vi "Edit Documentation of Properties.vi"   [LabVIEW 2015]
uses:
  Project Manipulation Scripts/Project Manipulation Scripts.lvlib
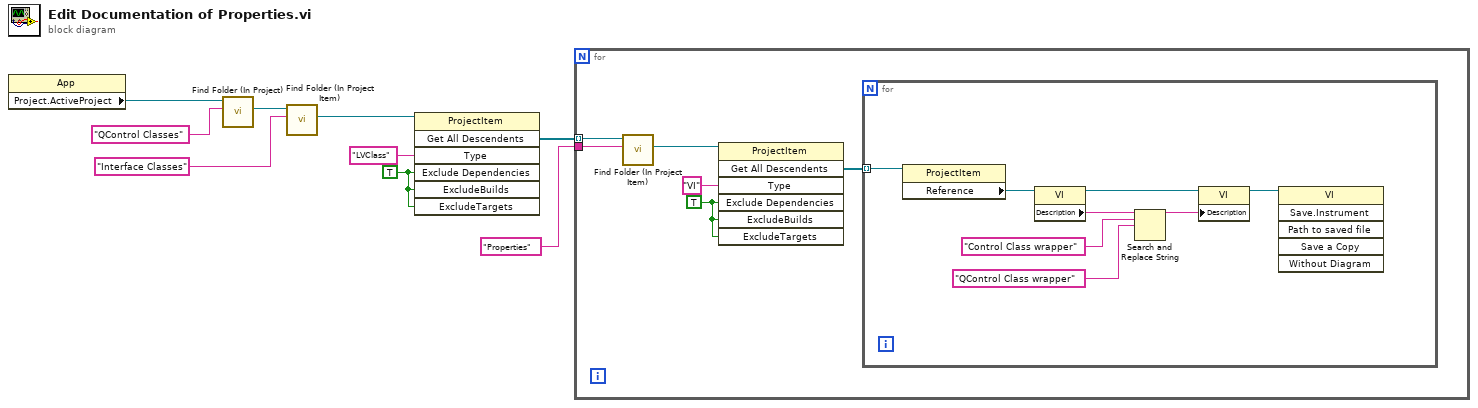
[diagram p0: block diagram]
diagram:
  w3 = TRUE ("ExcludeDependencies")
  n1 = property class="App"() -> ("Project.ActiveProject"=w8:refnum<vi>)  [unwired: 2 in, 2 out]
  n2 = call "Find Folder (In Project).vi"("Folder Name"="QControl Classes", "Project in"=w8) -> ("Folder Refnum"=w7:refnum<vi>)  [unwired: 7 in, 2 out]
  n3 = call "Find Folder (In Project Item).vi"("Folder Name"="Interface Classes", "ProjectItem in"=w7) -> ("Folder Refnum"=w4:refnum<vi>)  [unwired: 7 in, 2 out]
  n4 = invoke class="ProjectItem" method="Get All Descendents"(reference=w4, "Type"="LVClass", "Exclude Dependencies"=w3, "ExcludeBuilds"=w3, "ExcludeTargets"=w3) -> ("All Descendents"=w2:refnum<vi>[])  [unwired: 2 in, 6 out]
  n5 = for {
    tunnel: w2 -> [w15] mode=indexing
    tunnel: "Properties" ("Folder Name") -> [w14]
    w13 = TRUE ("ExcludeDependencies")
    n6 = call "Find Folder (In Project Item).vi"("Folder Name"=w14, "ProjectItem in"=w15) -> ("Folder Refnum"=w11:refnum<vi>)  [unwired: 7 in, 2 out]
    n7 = invoke class="ProjectItem" method="Get All Descendents"(reference=w11, "Type"="VI", "Exclude Dependencies"=w13, "ExcludeBuilds"=w13, "ExcludeTargets"=w13) -> ("All Descendents"=w10:refnum<vi>[])  [unwired: 2 in, 6 out]
    n8 = for {
      tunnel: w10 -> [w23] mode=indexing
      n9 = property class="ProjectItem"(reference=w23) -> ("Reference"=w22:refnum<vi>)  [unwired: 1 in, 2 out]
      n10 = property class="VI"(reference=w22) -> (reference out=w18:refnum<vi>, "Description"=w21:string)  [unwired: 1 in, 1 out]
      n11 = Search and Replace String(input string=w21, search string="Control Class wrapper", replace string="QControl Class wrapper" ("search string")) -> (result string=w17:string)  [unwired: 5 in, 3 out]
      n12 = property class="VI"(reference=w18, "Description"=w17) -> (reference out=w16:refnum<vi>)  [unwired: 1 in, 1 out]
      n13 = invoke class="VI" method="Save.Instrument"(reference=w16) -> ()  [unwired: 5 in, 6 out]
    }
  }
